vi "tutorial_11.vi"() -> ()   [LabVIEW 2021]
panel:
  out "Meter":dbl(knob) scale=0.0..100.0
  in  "On/off":bool
  in  "Knob":dbl(knob) scale=0.0..100.0
  in  "Temp Scale":bool
  out "Waveform Chart":cluster{dbl, "Thermometer":dbl}(graph)
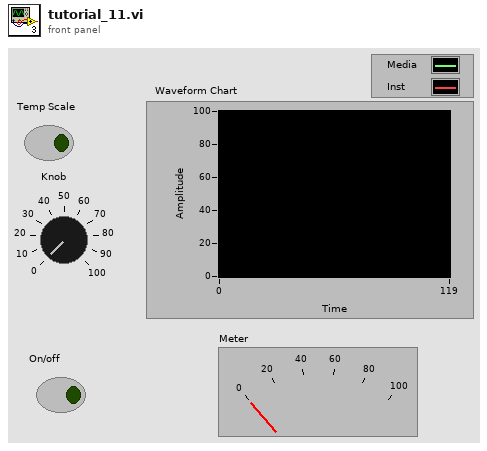
[diagram p1: front panel]
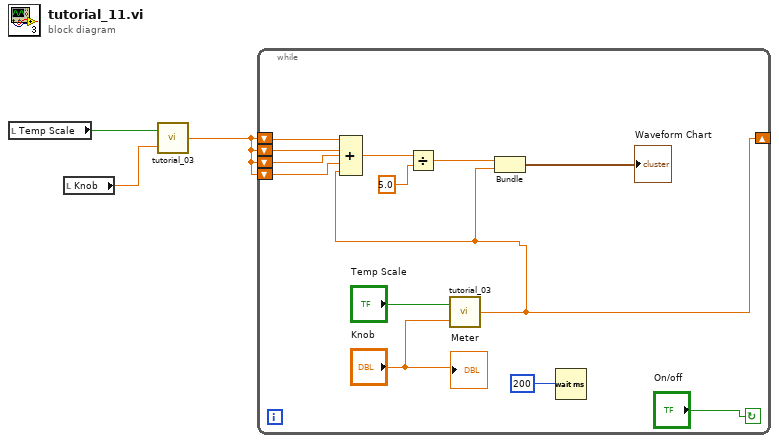
[diagram p0: block diagram]
diagram:
  n1 = local read "Temp Scale"() -> (w2:bool)
  n2 = local read "Knob"() -> (w1:dbl)
  n3 = call "tutorial_03.vi"("Knob"=w1, "Temp Scale"=w2) -> ("Thermometer"=w3:dbl)
  n4 = while {
    shift-right: [w4] -> _
    shift-left: w3 -> [w14]
    shift-left: w3 -> [w11]
    shift-left: w3 -> [w13]
    shift-left: w3 -> [w12]
    stop <- "On/off" continue-if-true
    n5 = call "tutorial_03.vi"("Knob"="Knob", "Temp Scale"="Temp Scale") -> ("Thermometer"=w4:dbl)
    n6 = Compound Arithmetic op=ADD(w14, w13, w12, w11, w4) -> (w10:dbl)
    n7 = Divide(x=w10, y=5.0 ("x/y")) -> (x/y=w8:dbl)
    n8 = Bundle(w8, "Thermometer"=w4) -> (→"Waveform Chart":cluster{dbl, "Thermometer":dbl})  [unwired: 1 in]
    n9 = Wait (ms)(milliseconds to wait=u32 200 ("millisecond timer value")) -> ()  [unwired: 1 out]
    "Meter" <- "Knob"
  }
